vi "Autocycle v0.2.vi"(7 "Message Queue":refnum<queue>, 8 "error in":errorcluster, 10 "Auto Para":T1={"Agitator Delays"=[], "TF Delays"=[], "Insertion Delays"=[], "Cutting Delays"=[], "PF Delays"=[], "Measur. Delays"=[1000.0], "Reject Delays"=[1000], "BF Delays"=[1000]}) -> (0 "error out":errorcluster)   [LabVIEW 2017]
uses:
  Controls/Auto Delays.ctl
  support/Message Queue/Message Cluster.ctl
  Controls/Auto Times.ctl
  Global Variables/RT GV.vi
  Global Variables/FPGA GV.vi
  <vilib>/Utility/error.llb/Error Cluster From Error Code.vi
  <vilib>/rvi/errors/niLvFpgaAdjustHostInterfaceError.vi
  support/Message Queue/Enqueue Message (Single).vi
  <vilib>/rvi/interface/nirviReadWriteControl/nirviReadWriteControl.xnode
  Controls/FPGA Ref.ctl
  NiFpgaLv.dll
  <vilib>/rvi/interface/Simulation/niFpgaSimulationCallBeginRW.vi
  support/Message Queue/Message Queue.lvlib
panel:
  in  "Max Successive":u32=5
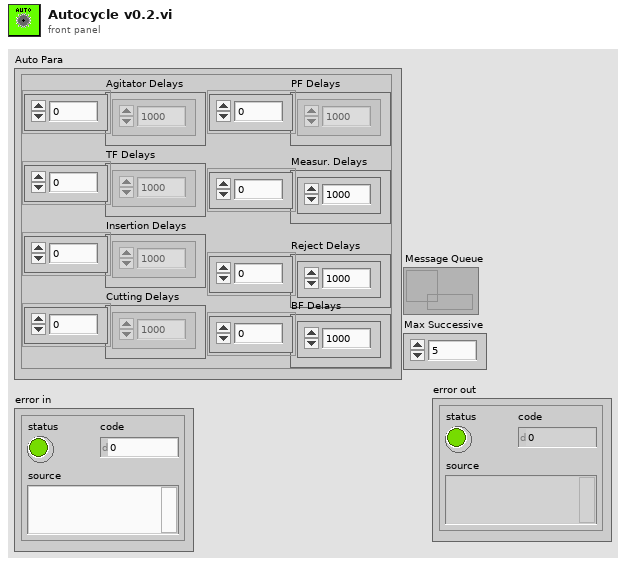
[diagram p1: front panel]
types:
  T1 = typedef "Auto Delays.ctl" = cluster{"Agitator Delays":u32[], "TF Delays":u32[], "Insertion Delays":u32[], "Cutting Delays":u32[], "PF Delays":u32[], "Measur. Delays":dbl[], "Reject Delays":u32[], "BF Delays":u32[]}
  T2 = cluster{"Tube Present":bool[], "Output Count":u32}
  T3 = typedef "FPGA Ref.ctl" = refnum<k20>
  T4 = cluster{"TL_Red":bool, "TL_Orange":bool, "TL_Green":bool, "TL_Buzzer":bool, "SOL_Index_Rotary_CW":bool, "SOL_Index_CNVR_Rotary_CCW":bool, "SOL_Index_CNVR_Stopper_Rear":bool, "SOL_Index_CNVR_Output _Separator _Rear":bool, "Bowl Feeder_ ON1":bool, "Pump_CNVR_Motor _ON":bool, "SOL_PC_Gating_CYL_Rear":bool, "SOL_Tube_Feed_Agitatator":bool, "SOL_Tube_Feed_Gating_CYL":bool, "SOL_Insertion _CYL":bool, "SOL_Insertion_Clamp_CYL":bool, "SOL_Cutting_CYL":bool, "SOL_Cutting_Clamp_CYL":bool, "SOL_Insertion_Air_Nozzle":bool, "SOL_Measurement_CYL":bool, "DO1.19":bool, "SOL_Rejection CYL_1":bool, "SOL_Rejection CYL_2":bool, "SOL_Rejection CYL_3":bool, "SOL_Rejection CYL_4":bool, "Bowl Feeder_ON2":bool, "SOL_BF_BlowerON":bool, "SOL_BF1_Track1":bool, "SOL_BF1_Track2":bool, "SOL_BF2_Track1":bool, "SOL_BF2_Track2":bool, "DO1.30":bool, "DO1.31":bool}
  T5 = typedef "Auto Times.ctl" = cluster{"Index Time":u32, "TF Time":u32, "Insertion Time":u32, "Cutting Time":u32, "PF Time":u32, "Meas. Time":u32, "Reject Time":u32}
  T6 = cluster{"Reject 1":bool, "Reject 2":bool, "Reject 3":bool, "Reject 4":bool}
  T7 = cluster{"Tube Present":bool[], "Parts Count":u32}
  T8 = cluster{"seconds since 1Jan1904":timestamp, "Auto Times":T5, "Parts Count":u32, "Reject Pallets":cluster{"Reject 1":bool, "Reject 2":bool, "Reject 3":bool, "Reject 4":bool}, "Measurements":cluster{"1":dbl, "2":dbl, "3":dbl, "4":dbl}}
  T9 = typedef "Auto Stats.ctl" = cluster{"Time-Stamp":timestamp, "Auto Times":T5, "Measurements":cluster{"1":dbl, "2":dbl, "3":dbl, "4":dbl}, "Outputs":cluster{"Good Parts":u32, "Reject Parts":u32}, "Cycle Time":dbl, "Remarks":string}
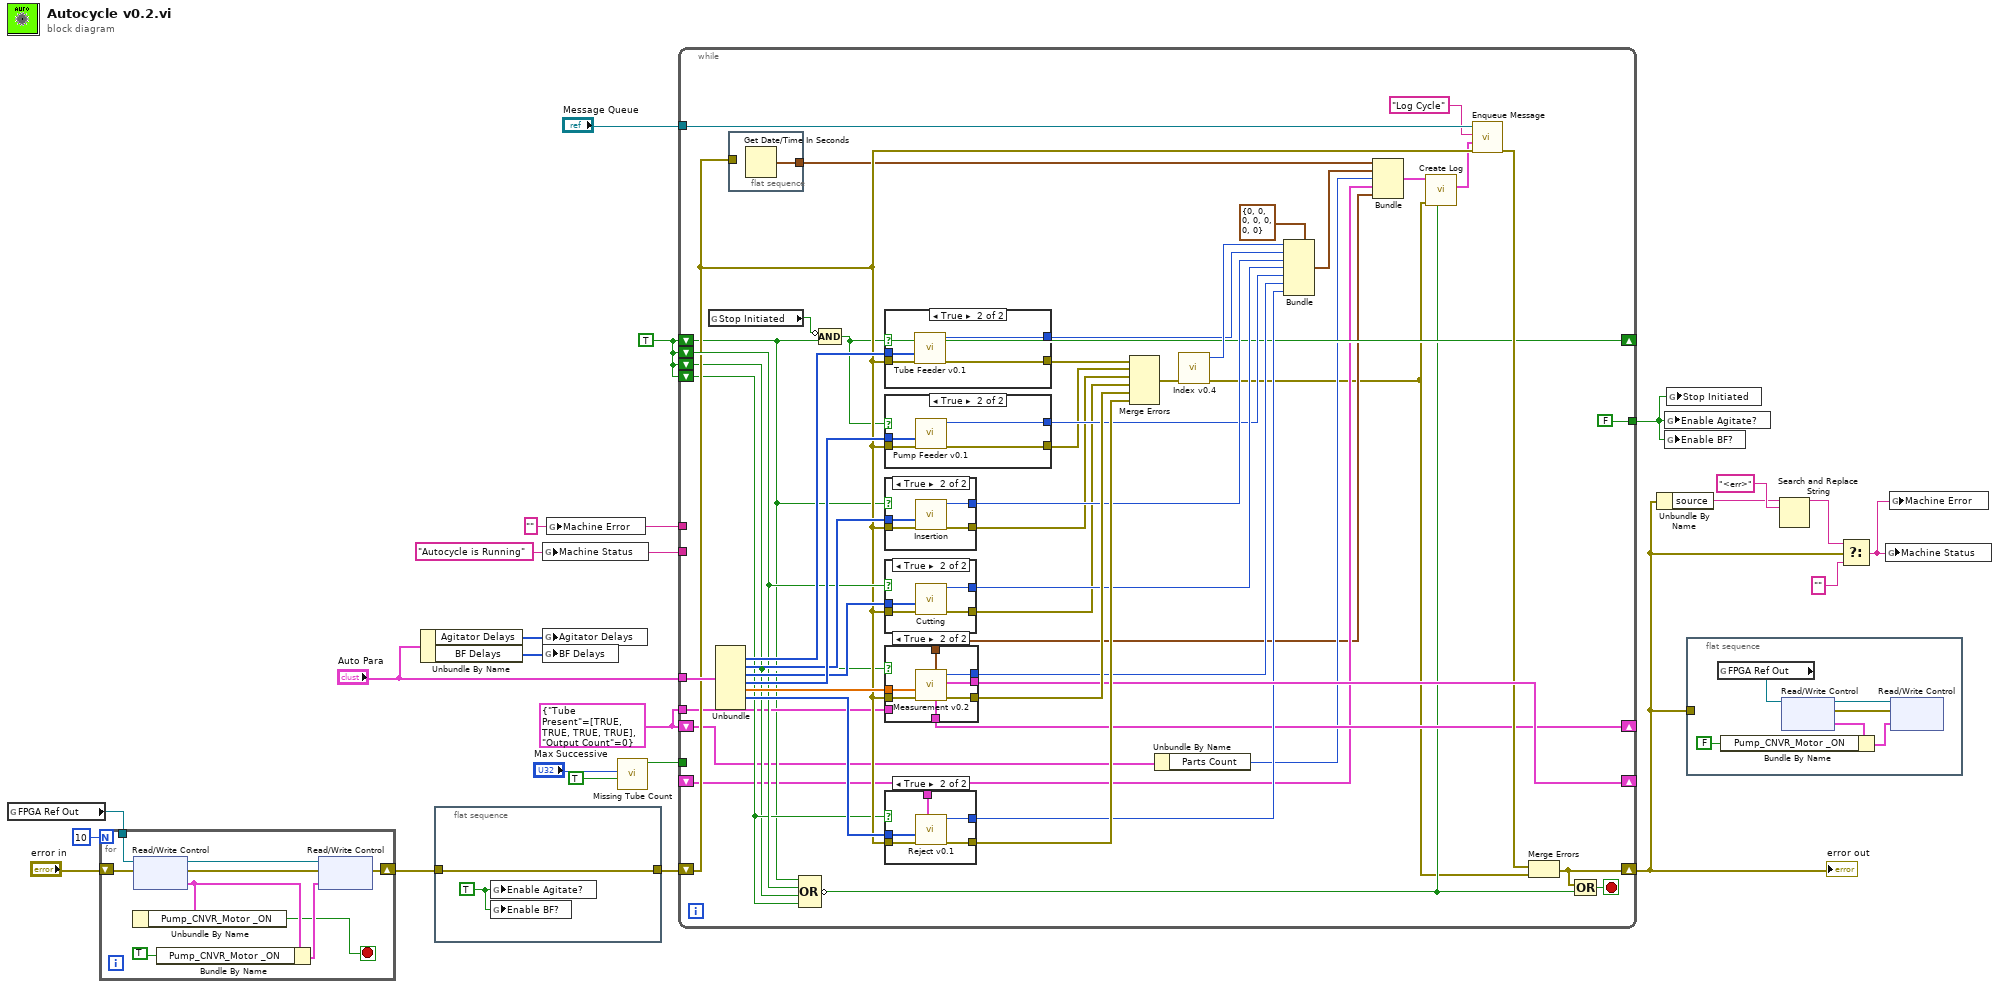
[diagram p0: block diagram]
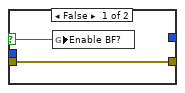
[diagram p2: hidden frame]
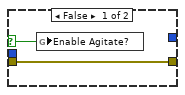
[diagram p5: hidden frame]
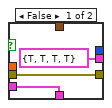
[diagram p7: hidden frame]
diagram:
  w7 = T2 {"Tube Present"=[TRUE, TRUE, TRUE, TRUE], "Output Count"=0} ("Part Count")
  w8 = "" ("Machine Error")
  w16 = "Autocycle is Running" ("Machine Status")
  w17 = TRUE
  n1 = global read "FPGA GV.vi" "FPGA Ref Out"() -> (w20:T3)
  n2 = for {
    N: 10 -> [_]
    tunnel: w20 -> [w32]
    shift-right: [w26] -> w3
    shift-left: "error in" -> [w27]
    stop <- w24 stop-if-true
    n3 = xnode "Read/Write Control"("FPGA VI Reference In"=w32, "error in"=w27) -> ("FPGA VI Reference Out"=w28:T3, "error out"=w29:errorcluster, "DO 1"=w25:T4)
    n4 = Unbundle By Name(w25) -> ("Pump_CNVR_Motor _ON"=w24:bool)
    n5 = Bundle By Name(cluster=w25, "Pump_CNVR_Motor _ON"=TRUE) -> (w31:T4)
    n6 = xnode "Read/Write Control"("FPGA VI Reference In"=w28, "error in"=w29, "DO 1"=w31) -> ("error out"=w26:errorcluster)  [unwired: 1 out]
  }
  n7 = Unbundle By Name("Auto Para") -> ("Agitator Delays"=w22:u32[], "BF Delays"=w21:u32[])
  n8 = flat-sequence {
    tunnel: [w34] -> w2
    tunnel: w3 -> [w34]
    frame #0 {
      w33 = TRUE ("Enable Agitate?")
      n9 = global write "RT GV.vi" "Enable Agitate?"(w33) -> ()
      n10 = global write "RT GV.vi" "Enable BF?"(w33) -> ()
    }
  }
  n11 = global write "RT GV.vi" "Machine Status"(w16) -> ()
  n12 = global write "RT GV.vi" "Agitator Delays"(w22) -> ()
  n13 = global write "RT GV.vi" "BF Delays"(w21) -> ()
  n14 = global write "RT GV.vi" "Machine Error"(w8) -> ()
  n15 = call "Missing Tube Count.vi"("ResetMT?"=TRUE, "Max Successive"="Max Successive") -> ("Boolean"=w4:bool)  [unwired: 9 in]
  n16 = while {
    tunnel: "Auto Para" -> [w78]
    shift-right: [w52] -> w14
    shift-left: w2 -> [w54]
    shift-right: [w72] -> _
    shift-left: _ -> [w39]
    shift-right: [w43] -> _
    shift-left: w17 -> [w42]
    shift-left: w17 -> [w55]
    shift-left: w17 -> [w49]
    shift-left: w17 -> [w50]
    tunnel: "Message Queue" -> [w61]
    tunnel: [FALSE] -> w10
    tunnel: w16 -> [_]
    tunnel: w8 -> [_]
    shift-right: [w44] -> _
    shift-left: w7 -> [w41]
    tunnel: w7 -> [w45]
    tunnel: w4 -> [_]
    stop <- w71 stop-if-true
    n17 = global read "RT GV.vi" "Stop Initiated"() -> (w62:bool)
    n18 = Unbundle(w78) -> ("TF Delays"=w81:u32[], "Insertion Delays"=w80:u32[], "Cutting Delays"=w79:u32[], "PF Delays"=w82:u32[], "Measur. Delays"=w76:dbl[], "Reject Delays"=w74:u32[])  [unwired: 2 out]
    n19 = flat-sequence {
      tunnel: w54 -> [_]
      tunnel: [w83] -> w47
      frame #0 {
        n20 = Get Date/Time In Seconds() -> (seconds since 1Jan1904=w83:timestamp)
      }
    }
    n21 = Compound Arithmetic op=OR(w42, w55, w49, w50) -> (invert w37:bool)
    n22 = Compound Arithmetic op=AND(invert w62, w42) -> (w43:bool)
    n23 = case shown="True" w43 {
      selector: w43 -> [w100 _]
      tunnel: w54 -> [w101 w105]
      tunnel: [w101 w104] -> w77
      tunnel: w81 -> [_ w103]
      tunnel: [_ w102] -> w69
      frame False {
        n24 = global write "RT GV.vi" "Enable Agitate?"(w100) -> ()
      }
      frame True {
        n25 = call "Tube Feeder v0.1.vi"("error in (no error)"=w105, "TF Para"=w103) -> ("error out"=w104:errorcluster, "TF Time"=w102:u32)  [unwired: 8 in]
      }
    }
    n26 = case shown="True" w43 {
      selector: w43 -> [w84 _]
      tunnel: w54 -> [w85 w89]
      tunnel: [w85 w88] -> w57
      tunnel: w82 -> [_ w87]
      tunnel: [_ w86] -> w66
      frame False {
        n27 = global write "RT GV.vi" "Enable BF?"(w84) -> ()
      }
      frame True {
        n28 = call "Pump Feeder v0.1.vi"("error in (no error)"=w89, "TF Delays"=w87) -> ("error out"=w88:errorcluster, "PF Time"=w86:u32)  [unwired: 8 in]
      }
    }
    n29 = case shown="True" w42 {
      tunnel: w54 -> [w95 w99]
      tunnel: [w95 w98] -> w58
      tunnel: w80 -> [_ w97]
      tunnel: [_ w96] -> w68
      frame False {
      }
      frame True {
        n30 = call "Insertion.vi"("error in (no error)"=w99, "Insertion Delays"=w97) -> ("error out"=w98:errorcluster, "Insertion Time"=w96:u32)  [unwired: 7 in, 1 out]
      }
    }
    n31 = case shown="True" w55 {
      tunnel: w54 -> [w90 w94]
      tunnel: [w90 w93] -> w59
      tunnel: w79 -> [_ w92]
      tunnel: [_ w91] -> w67
      frame False {
      }
      frame True {
        n32 = call "Cutting.vi"("error in (no error)"=w94, "Cutting Delays"=w92) -> ("error out"=w93:errorcluster, "Cutting Time"=w91:u32)  [unwired: 8 in]
      }
    }
    n33 = case shown="True" w49 {
      tunnel: w54 -> [w114 w121]
      tunnel: [w114 w120] -> w75
      tunnel: w76 -> [_ w119]
      tunnel: [_ w118] -> w65
      tunnel: [_ w117] -> w38
      tunnel: [T6 {"Reject 1"=TRUE, "Reject 2"=TRUE, "Reject 3"=TRUE, "Reject 4"=TRUE} ("Reject Pallets") w116] -> w72
      tunnel: [w112 w115] -> w44
      tunnel: w45 -> [w112 _]
      frame False {
      }
      frame True {
        n34 = call "Measurement v0.2.vi"("error in (no error)"=w121, "TF Delays"=w119) -> ("error out"=w120:errorcluster, "Reject Pallets"=w116:T6, "PF Time"=w118:u32, "Part Count"=w115:T7, "Measurements"=w117:cluster{"1":dbl, "2":dbl, "3":dbl, "4":dbl})  [unwired: 5 in]
      }
    }
    n35 = case shown="True" w50 {
      tunnel: w54 -> [w106 w111]
      tunnel: [w106 w110] -> w73
      tunnel: w74 -> [_ w109]
      tunnel: [_ w108] -> w64
      tunnel: w39 -> [_ w107]
      frame False {
      }
      frame True {
        n36 = call "Reject v0.1.vi"("Reject Pallets"=w107, "error in (no error)"=w111, "TF Delays"=w109) -> ("error out"=w110:errorcluster, "PF Time"=w108:u32)  [unwired: 7 in]
      }
    }
    n37 = Merge Errors(w77, w57, w58, w59, w75, w73) -> (w53:errorcluster)
    n38 = Unbundle By Name(w41) -> ("Parts Count"=w40:u32)
    n39 = call "Index v0.4.vi"("error in (no error)"=w53) -> ("error out"=w35:errorcluster, "Index Time"=w70:u32)  [unwired: 7 in, 2 out]
    n40 = Bundle(cluster=T5 {"Index Time"=0, "TF Time"=0, "Insertion Time"=0, "Cutting Time"=0, "PF Time"=0, "Meas. Time"=0, "Reject Time"=0} ("Auto Times"), "Index Time"=w70, "TF Time"=w69, "Insertion Time"=w68, "Cutting Time"=w67, "PF Time"=w66, "Meas. Time"=w65, "Reject Time"=w64) -> (w46:T5)
    n41 = Bundle("seconds since 1Jan1904"=w47, "Auto Times"=w46, "Parts Count"=w40, "Reject Pallets"=w39, "Measurements"=w38) -> (w36:T8)  [unwired: 1 in]
    n42 = call "Create Log.vi"("Stopped"=w37, "Error in"=w35, "Log Input Data"=w36) -> ("Auto Stats"=w48:T9)  [unwired: 8 in]
    n43 = call-poly "Enqueue Message.vi"("error in (no error)"=w54, "Message Data"=w48, "Message"="Log Cycle", "Message Queue"=w61) -> ("error out"=w51:errorcluster)  [unwired: 6 in, 1 out]
    n44 = Merge Errors(w51, w35) -> (w52:errorcluster)
    n45 = Compound Arithmetic op=OR(w52, w37) -> (w71:bool)
  }
  "error out" <- w14
  n46 = Unbundle By Name(w14) -> ("source"=w12:string)
  n47 = global write "RT GV.vi" "Enable Agitate?"(w10) -> ()
  n48 = global write "RT GV.vi" "Enable BF?"(w10) -> ()
  n49 = global write "RT GV.vi" "Stop Initiated"(w10) -> ()
  n50 = flat-sequence {
    tunnel: w14 -> [_]
    frame #0 {
      n51 = global read "FPGA GV.vi" "FPGA Ref Out"() -> (w122:T3)
      n52 = xnode "Read/Write Control"("FPGA VI Reference In"=w122) -> ("FPGA VI Reference Out"=w127:T3, "error out"=w126:errorcluster, "DO 1"=w124:T4)  [unwired: 1 in]
      n53 = Bundle By Name(cluster=w124, "Pump_CNVR_Motor _ON"=FALSE) -> (w125:T4)
      n54 = xnode "Read/Write Control"("FPGA VI Reference In"=w127, "error in"=w126, "DO 1"=w125) -> ()  [unwired: 2 out]
    }
  }
  n55 = Search and Replace String(input string=w12, search string="<err>") -> (result string=w11:string)  [unwired: 6 in, 3 out]
  n56 = Select(t=w11, s=w14, f="" ("Machine Status")) -> (s? t:f=w9:string)
  n57 = global write "RT GV.vi" "Machine Status"(w9) -> ()
  n58 = global write "RT GV.vi" "Machine Error"(w9) -> ()
